vi "Calculate Indices.vi"(1 "Linked? Array":bool[](array[boolean]), 2 "Index of script":i32=1, 3 "Sizes of Arrays":i32[](array[numeric])) -> (0 "Indices":i32[](array[numeric]))   [LabVIEW 2020, in "CIRCUS_uServices.lvlib" / "Run Utilities.lvlib" / "Scan SBlock.lvclass"]
doc: "Creates an array of indices for each paramter based on the iterator value"
uses:
  Scan SBlock.lvclass
  Scan SBlock.lvclass/Scan SBlock.ctl
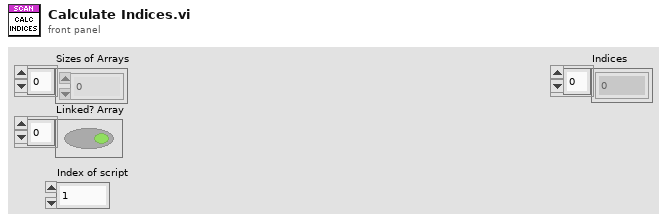
[diagram p1: front panel]
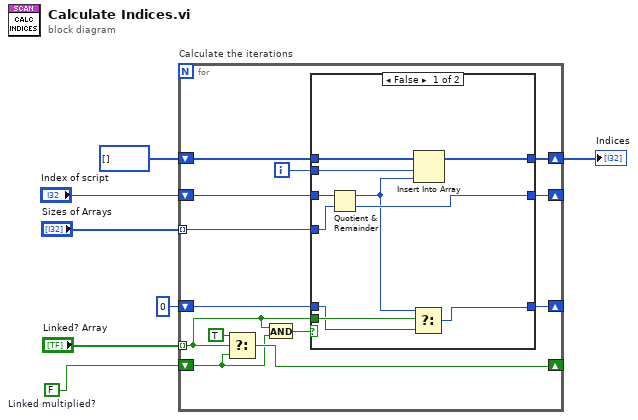
[diagram p0: block diagram]
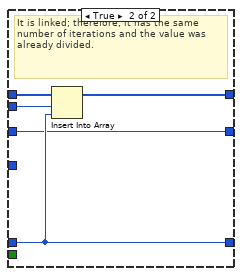
[diagram p2: hidden frame]
diagram:
  w6 = FALSE  # Linked multiplied?
  n1 = for "Calculate the iterations" {
    tunnel: "Sizes of Arrays" -> [w15] mode=indexing
    shift-right: [w9] -> _
    shift-left: "Index of script" -> [w16]
    tunnel: "Linked? Array" -> [w8] mode=indexing
    shift-right: [w19] -> _
    shift-left: w6 -> [w18]
    shift-right: [w10] -> w2
    shift-left: i32[] [] ("array") -> [w13]
    shift-right: [w12] -> _
    shift-left: 0 -> [w11]
    i -> [w14]
    n2 = Select(t=TRUE, s=w8, f=w18) -> (s? t:f=w19:bool)
    n3 = And(x=w8, y=w18) -> (x .and. y?=w17:bool)
    n4 = case shown="False" w17 {
      tunnel: w16 -> [w28 w31]
      tunnel: w15 -> [w27 _]
      tunnel: w14 -> [w21 w33]
      tunnel: w13 -> [w30 w35]
      tunnel: [w23 w34] -> w12
      tunnel: w11 -> [w24 w34]
      tunnel: [w29 w32] -> w10
      tunnel: [w26 w31] -> w9
      tunnel: w8 -> [w25 _]
      frame False {
        n5 = Quotient & Remainder(x=w28, y=w27) -> (x-y*floor(x/y)=w22:i32, floor(x/y)=w26:i32)
        n6 = Select(t=w22, s=w25, f=w24) -> (s? t:f=w23:i32)
        n7 = Insert Into Array(array=w30, index=w21, new element=w22) -> (w29:i32[])
      }
      frame True {
        # "It is linked; therefore, it has the same number of iterations and the value was already divided."
        n8 = Insert Into Array(array=w35, index=w33, new element=w34) -> (w32:i32[])
      }
    }
  }
  "Indices" <- w2
